vi "Tools_Windows Memory Status.vi"(8 "error in (no error)":errorcluster) -> (0 "error out":errorcluster, 1 "Free memory (%)":dbl, 2 "Free memory (KB)":dbl format="%#_6f", 3 "Total memory (KB)":dbl format="%#_6f")   [LabVIEW 2014]
uses:
  kernel32.dll
panel:
  out "Total memory (MB)":dbl
  out "Free memory (MB)":dbl
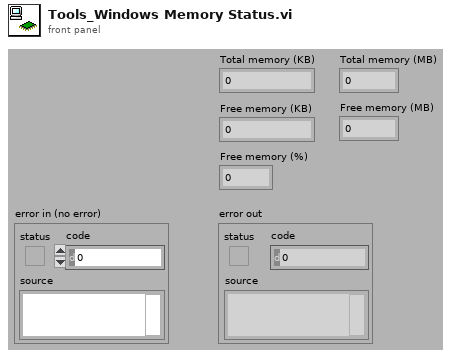
[diagram p1: front panel]
types:
  T1 = cluster{"dwLength":u32, "dwMemoryLoad":u32, "ullTotalPhys":u64, "ullAvailPhys":u64, "ullTotalPageFile":u64, "ullAvailPageFile":u64, "ullTotalVirtual":u64, "ullAvailVirtual":u64, "ullAvailExtendedVirtual":u64}
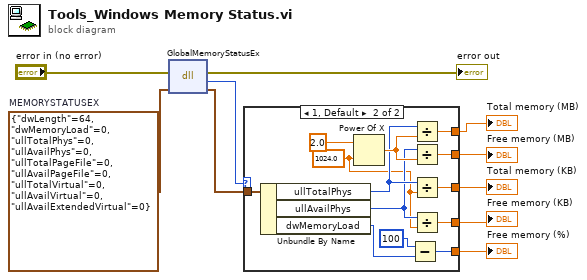
[diagram p0: block diagram]
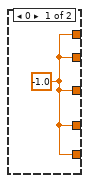
[diagram p2: hidden frame]
diagram:
  w5 = T1 {"dwLength"=64, "dwMemoryLoad"=0, "ullTotalPhys"=0, "ullAvailPhys"=0, "ullTotalPageFile"=0, "ullAvailPageFile"=0, "ullTotalVirtual"=0, "ullAvailVirtual"=0, "ullAvailExtendedVirtual"=0}  # MEMORYSTATUSEX
  n1 = dll-call lib="kernel32.dll" fn="GlobalMemoryStatusEx"(error in="error in (no error)", w5) -> (error out=→"error out":errorcluster, "return type"=w6:i32, w7:T1)  [unwired: 2 in, 1 out]
  n2 = case shown="1, Default" w6 {
    tunnel: w7 -> [_ w24]
    tunnel: [w11 w19] -> w10
    tunnel: [w11 w16] -> w8
    tunnel: [w11 w15] -> w9
    tunnel: [w11 w18] -> w2
    tunnel: [w11 w17] -> w1
    frame 0 {
      w11 = -1.0
    }
    frame 1, Default {
      w12 = 1024.0 ("x")
      n3 = Unbundle By Name(w24) -> ("ullTotalPhys"=w14:u64, "ullAvailPhys"=w13:u64, "dwMemoryLoad"=w20:u32)
      n4 = Power Of X(1:w12, 2:2.0 ("y")) -> (0:w22:dbl)
      n5 = Subtract(x=u32 100, y=w20) -> (x-y=w19:u32)
      n6 = Divide(x=w14, y=w22) -> (x/y=w18:dbl)
      n7 = Divide(x=w13, y=w22) -> (x/y=w17:dbl)
      n8 = Divide(x=w14, y=w12) -> (x/y=w16:dbl)
      n9 = Divide(x=w13, y=w12) -> (x/y=w15:dbl)
    }
  }
  "Free memory (%)" <- w10
  "Free memory (KB)" <- w9
  "Total memory (KB)" <- w8
  "Free memory (MB)" <- w1
  "Total memory (MB)" <- w2
